vi "Size Menu to Screen.vi"(8 "error IO":errorcluster, 11 "User Interface References":T1) -> (0 "error out":errorcluster, 3 "User Interface References Out":T1={"This VI"=refnum, "User Interace Plugin"=refnum, "UI Picture Container References"={"Header Image"=refnum, "Footer Image"=refnum}, "Sliding Menu XControl"=refnum, "Menu Container"=refnum, "UI Configuration Information"={"Space Between Buttons"=3, "Number of Buttons to Show"=6, "Header Image"=path "Images/Blue Background.bmp", "Footer Image"=path "Images/Blue Background.bmp"}, "Header Text"=refnum})   [LabVIEW 2011]
uses:
  Main Type Definitions/User Interface Type Definitions.ctl
  Sliding Menu/Sliding Menu Library/Sliding Menu SubVIs/Sliding Menu Type Definitions/UI Picture Containers.ctl
  Sliding Menu/Sliding Menu Library/Sliding Menu xControl/Sliding Menu XControl.xctl
  UI Control Definitions/UI Configuration Information.ctl
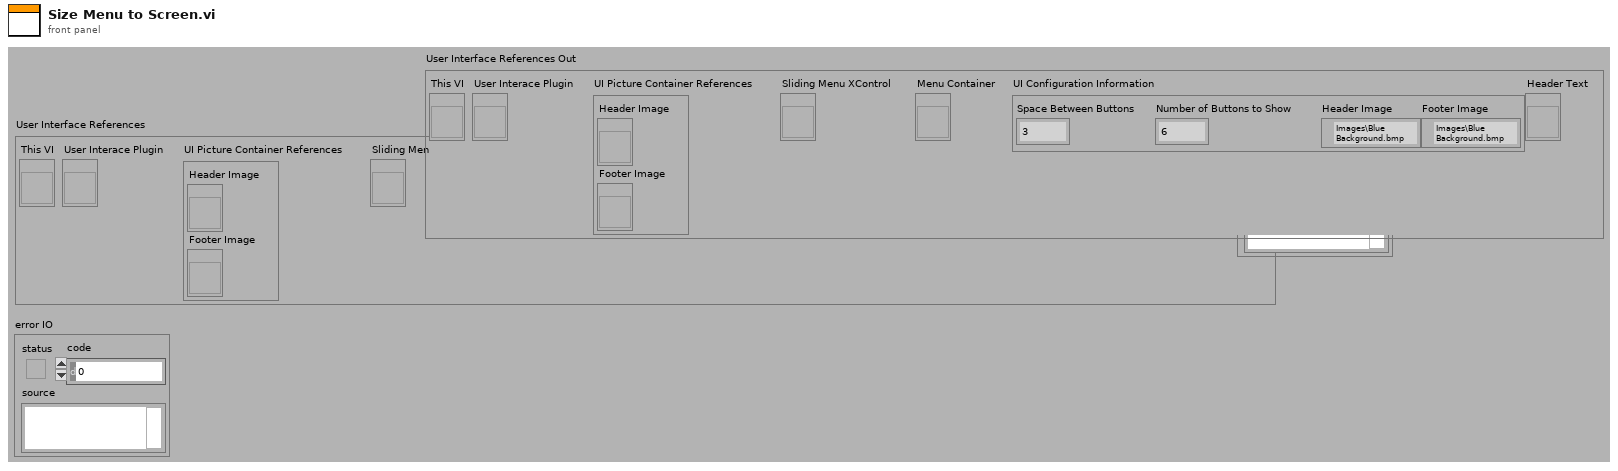
[diagram p1: front panel]
types:
  T1 = typedef "User Interface Type Definitions.ctl" = cluster{"This VI":refnum<vi>, "User Interace Plugin":refnum<vi>, "UI Picture Container References":T2, "Sliding Menu XControl":refnum<vi>, "Menu Container":refnum<vi>, "UI Configuration Information":T3, "Header Text":refnum<vi>}
  T2 = typedef "UI Picture Containers.ctl" = cluster{"Header Image":refnum<vi>, "Footer Image":refnum<vi>}
  T3 = typedef "UI Configuration Information.ctl" = cluster{"Space Between Buttons":i32, "Number of Buttons to Show":i32, "Header Image":path, "Footer Image":path}
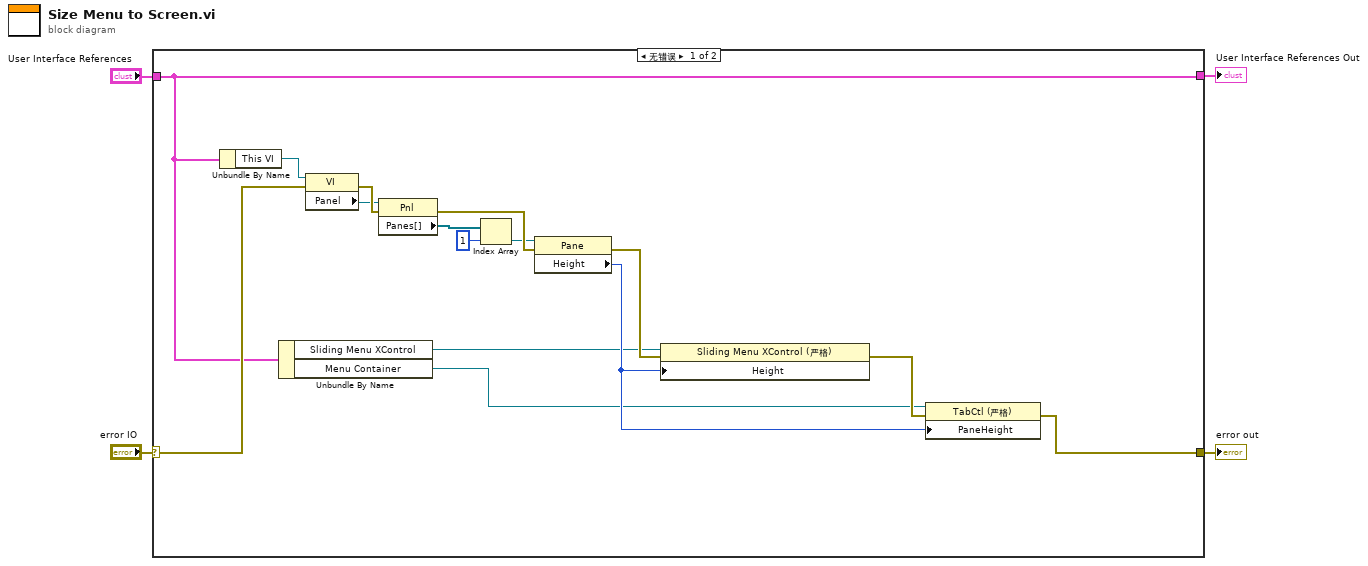
[diagram p0: block diagram]
diagram:
  n1 = case shown="无错误" "error IO" {
    selector: "error IO" -> [w6 w20]
    tunnel: "User Interface References" -> [w5 w21]
    tunnel: [w19 w20] -> w3
    tunnel: [w5 w21] -> w1
    frame No Error {
      n2 = Unbundle By Name(w5) -> ("This VI"=w7:refnum<vi>)
      n3 = Unbundle By Name(w5) -> ("Sliding Menu XControl"=w12:refnum<vi>, "Menu Container"=w13:refnum<vi>)
      n4 = property class="VI"(reference=w7, error in=w6) -> (error out=w18:errorcluster, "Panel"=w8:refnum<vi>)  [unwired: 1 out]
      n5 = property class="Pnl"(reference=w8, error in=w18) -> (error out=w17:errorcluster, "Panes[]"=w9:refnum<vi>[])  [unwired: 1 out]
      n6 = Index Array(array=w9, index=1) -> (element=w11:refnum<vi>)
      n7 = property class="Pane"(reference=w11, error in=w17) -> (error out=w16:errorcluster, "Height"=w14:u32)  [unwired: 1 out]
      n8 = property class="Sliding Menu XControl (严格)"(reference=w12, error in=w16, "Height"=w14) -> (error out=w15:errorcluster)  [unwired: 1 out]
      n9 = property class="TabCtl (严格)"(reference=w13, error in=w15, "PaneHeight"=w14) -> (error out=w19:errorcluster)  [unwired: 1 out]
    }
    frame Error {
    }
  }
  "error out" <- w3
  "User Interface References Out" <- w1
